vi "device in.vi"(0 "handle":i32) -> (8 "maxVelocityThreeAxis":dbl, 9 "Out":string, 10 "minVelocity":dbl, 11 "Firmware Version":i16, 12 "serialNumber":i32, 13 "maxVelocityTwoAxis":dbl, 14 "Dll Version":i16, 15 "DLL Revision":i16, 16 "encoderResolution":dbl, 17 "Firmware Profile":i16, 18 "stepSize":dbl, 19 "maxVelocity":dbl)   [LabVIEW 2012]
uses:
  MicroDrive.dll
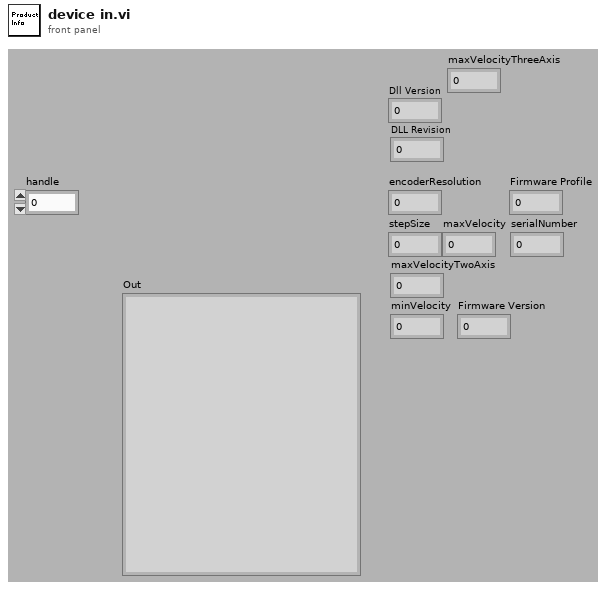
[diagram p1: front panel]
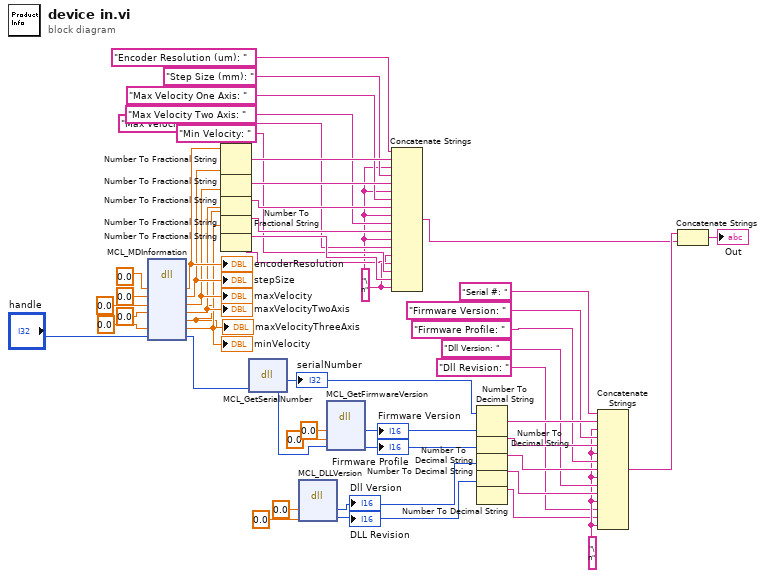
[diagram p0: block diagram]
diagram:
  w12 = "\n" ("F-format string")
  w1 = "\n" ("F-format string")
  n1 = dll-call lib="C:/Users/Labview/Desktop/SRR/MicroDrive_x64/Labview Examples/MicroDrive.dll" fn="MCL_MDInformation"("encoderResolution"=0.0, "stepSize"=0.0, "maxVelocity"=0.0, "maxVelocityTwoAxis"=0.0, "minVelocity"=0.0, "handle"="handle") -> ("encoderResolution"=w40:dbl, "stepSize"=w39:dbl, "maxVelocity"=w38:dbl, "maxVelocityTwoAxis"=w37:dbl, "maxVelocityThreeAxis"=w4:dbl, "minVelocity"=w36:dbl, "handle"=w27:i32)  [unwired: 3 in, 4 out]
  "encoderResolution" <- w40
  "stepSize" <- w39
  "maxVelocity" <- w38
  "maxVelocityTwoAxis" <- w37
  "minVelocity" <- w36
  "maxVelocityThreeAxis" <- w4
  n2 = Number To Fractional String(number=w40) -> (F-format string=w34:string)  [unwired: 3 out]
  n3 = Number To Fractional String(number=w39) -> (F-format string=w32:string)  [unwired: 3 out]
  n4 = Number To Fractional String(number=w38) -> (F-format string=w30:string)  [unwired: 3 out]
  n5 = Number To Fractional String(number=w37) -> (F-format string=w28:string)  [unwired: 3 out]
  n6 = Number To Fractional String(number=w4) -> (F-format string=w3:string)  [unwired: 3 out]
  n7 = Number To Fractional String(number=w36) -> (F-format string=w6:string)  [unwired: 3 out]
  n8 = dll-call lib="C:/Users/Labview/Desktop/SRR/MicroDrive_x64/Labview Examples/MicroDrive.dll" fn="MCL_GetSerialNumber"("handle"=w27) -> ("serialNumber"=w25:i32, "handle"=w26:i32)  [unwired: 3 in, 2 out]
  "serialNumber" <- w25
  n9 = dll-call lib="C:/Users/Labview/Desktop/SRR/MicroDrive_x64/Labview Examples/MicroDrive.dll" fn="MCL_DLLVersion"("version"=sgl 0.0, "revision"=sgl 0.0) -> ("version"=w22:i16, "revision"=w21:i16)  [unwired: 3 in, 3 out]
  "Dll Version" <- w22
  "DLL Revision" <- w21
  n10 = dll-call lib="C:/Users/Labview/Desktop/SRR/MicroDrive_x64/Labview Examples/MicroDrive.dll" fn="MCL_GetFirmwareVersion"("version"=sgl 0.0, "profile"=sgl 0.0, "handle"=w26) -> ("version"=w24:i16, "profile"=w23:i16)  [unwired: 4 in, 3 out]
  "Firmware Version" <- w24
  "Firmware Profile" <- w23
  n11 = Concatenate Strings("Encoder Resolution (um): " ("F-format string"), w34, w1, "Step Size (mm): " ("F-format string"), w32, w1, "Max Velocity One Axis: " ("F-format string"), w30, w1, "Max Velocity Two Axis: " ("F-format string"), w28, w1, "Max Velocity Three Axis: " ("F-format string"), w3, w1, "Min Velocity: " ("F-format string"), w6, w1) -> (w8:string)
  n12 = Number To Decimal String(number=w25) -> (decimal integer string=w19:string)  [unwired: 1 out]
  n13 = Number To Decimal String(number=w24) -> (decimal integer string=w17:string)  [unwired: 1 out]
  n14 = Number To Decimal String(number=w23) -> (decimal integer string=w15:string)  [unwired: 1 out]
  n15 = Number To Decimal String(number=w22) -> (decimal integer string=w13:string)  [unwired: 1 out]
  n16 = Number To Decimal String(number=w21) -> (decimal integer string=w11:string)  [unwired: 1 out]
  n17 = Concatenate Strings("Serial #: " ("F-format string"), w19, w12, "Firmware Version: " ("F-format string"), w17, w12, "Firmware Profile: " ("F-format string"), w15, w12, "Dll Version: " ("F-format string"), w13, w12, "Dll Revision: " ("F-format string"), w11, w12) -> (w9:string)
  n18 = Concatenate Strings(w9, w8) -> (→"Out":string)
